vi "[Generate Test Cases] Strip path.vi"() -> (3 "Strip path test cases":refnum<class "TestCase.lvclass">[](array[class]))   [LabVIEW 2015, in "Tests.lvlib" / "[Test Suite] File Transfer Helpers.lvclass"]
uses:
  [Test Suite] File Transfer Helpers.lvclass
  <vilib>/addons/_JKI Toolkits/VI Tester/TestCase.llb/TestCase.lvclass
  [Test Case] Fix Path/[Test Case] Fix path.lvclass
  [Test Case] Strip path/[Test Case] Strip path.lvclass
  [Test Case] Strip path/[Test Case] Strip path.lvclass/[Test Case] Strip path.ctl
  [Test Case] Strip path/Write Path in.vi
  [Test Case] Strip path/Write Expected stripped path.vi
  [Test Case] Strip path/Write Expected name.vi
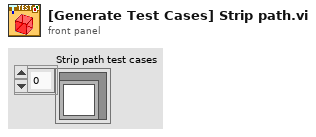
[diagram p1: front panel]
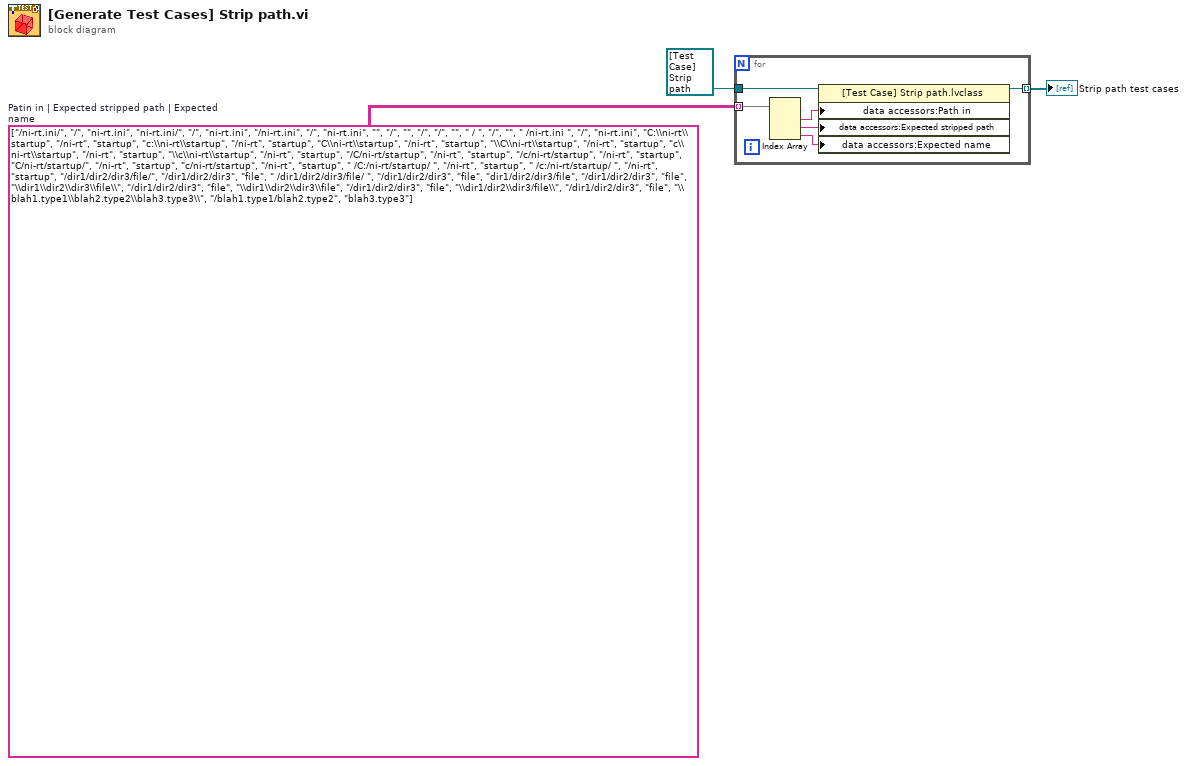
[diagram p0: block diagram]
diagram:
  w2 = string[][] [["/ni-rt.ini/", "/", "ni-rt.ini"], ["ni-rt.ini/", "/", "ni-rt.ini"], ["/ni-rt.ini", "/", "ni-rt.ini"], ["", "/", ""], ["/", "/", ""], [" / ", "/", ""], [" /ni-rt.ini ", "/", "ni-rt.ini"], ["C:\\ni-rt\\startup", "/ni-rt", "startup"], ["c:\\ni-rt\\startup", "/ni-rt", "startup"], ["C\\ni-rt\\startup", "/ni-rt", "startup"], ["\\C\\ni-rt\\startup", "/ni-rt", "startup"], ["c\\ni-rt\\startup", "/ni-rt", "startup"], ["\\c\\ni-rt\\startup", "/ni-rt", "startup"], ["/C/ni-rt/startup", "/ni-rt", "startup"], ["/c/ni-rt/startup", "/ni-rt", "startup"], ["C/ni-rt/startup/", "/ni-rt", "startup"], ["c/ni-rt/startup", "/ni-rt", "startup"], [" /C:/ni-rt/startup/ ", "/ni-rt", "startup"], [" /c:/ni-rt/startup/ ", "/ni-rt", "startup"], ["/dir1/dir2/dir3/file/", "/dir1/dir2/dir3", "file"], [" /dir1/dir2/dir3/file/ ", "/dir1/dir2/dir3", "file"], ["dir1/dir2/dir3/file", "/dir1/dir2/dir3", "file"], ["\\dir1\\dir2\\dir3\\file\\", "/dir1/dir2/dir3", "file"], ["\\dir1\\dir2\\dir3\\file", "/dir1/dir2/dir3", "file"], ["\\dir1/dir2\\dir3/file\\", "/dir1/dir2/dir3", "file"], ["\\blah1.type1\\blah2.type2\\blah3.type3\\", "/blah1.type1/blah2.type2", "blah3.type3"]]  # Patin in | Expected stripped path | Expected name
  n1 = for {
    tunnel: refnum<class "[Test Case] Strip path.lvclass"> refnum ("[Test Case] Fix Path.lvclass") -> [w9]
    tunnel: [w8] -> w1 mode=indexing
    tunnel: w2 -> [w7] mode=indexing
    n2 = Index Array(array=w7) -> (element #1=w6:string, element #2=w5:string, element #3=w4:string)  [unwired: 3 in]
    n3 = property class="[Test Case] Strip path.lvclass"(reference=w9, "data accessors:Path in"=w6, "data accessors:Expected stripped path"=w5, "data accessors:Expected name"=w4) -> (reference out=w8:refnum<class "[Test Case] Strip path.lvclass">)  [unwired: 1 in, 1 out]
  }
  "Strip path test cases" <- w1
